vi "Assign DRT values from string.vi"(1 "Syntax":enum16{"GCS 1.0", "GCS 2.0"}(ring), 2 "Queried axes":string[](array[string]), 3 "Parameter no.":i32[](array[numeric]), 4 "Input string":string, 5 "error in":errorcluster, 6 "Parameter no. (hex)":u32[](array[numeric]) format="%.0x", 7 "Parameter no. format \n(Decimal: FALSE)":bool) -> (11 "Parameter no. out":i32[](array[numeric]), 12 "Queried axes out":string[](array[string]), 13 "Parameter no. (hex) out":u32[](array[numeric]) format="%.0x", 14 "Parameter values":dbl[](array[numeric]) format="%.6f", 15 "Parameter strings":string[](array[string]), 19 "error out":errorcluster)   [LabVIEW 2020]
doc: "This VI assigns numerical values / strings from input string to queried axes and parameter numbers. Sub-VI for DRT?.vi."
panel:
  # "This vi assigns values/strings from input string to queried axes and parameter numbers."
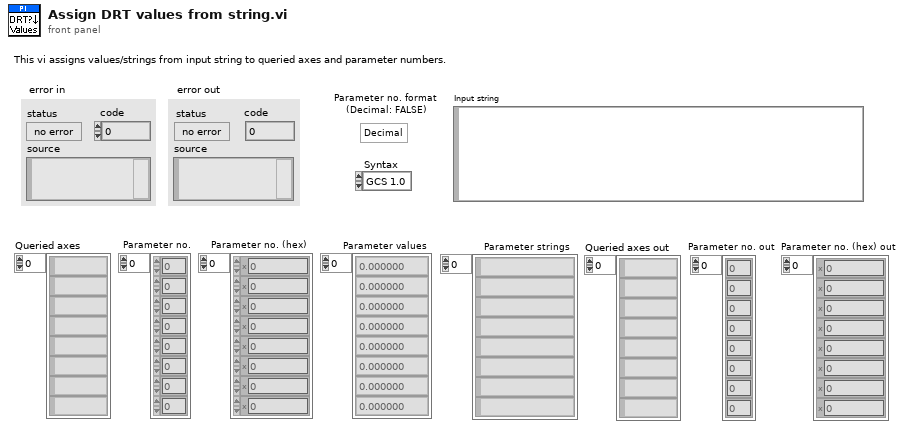
[diagram p1: front panel]
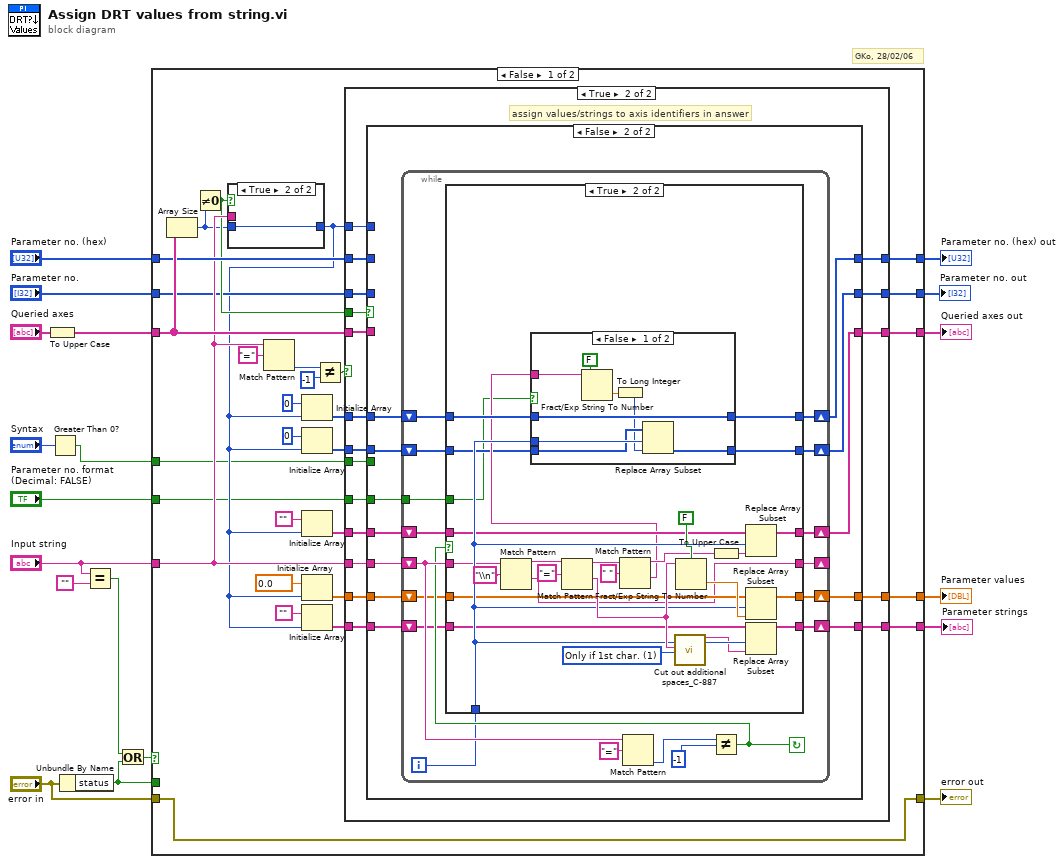
[diagram p0: block diagram]
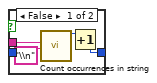
[diagram p2: hidden frame]
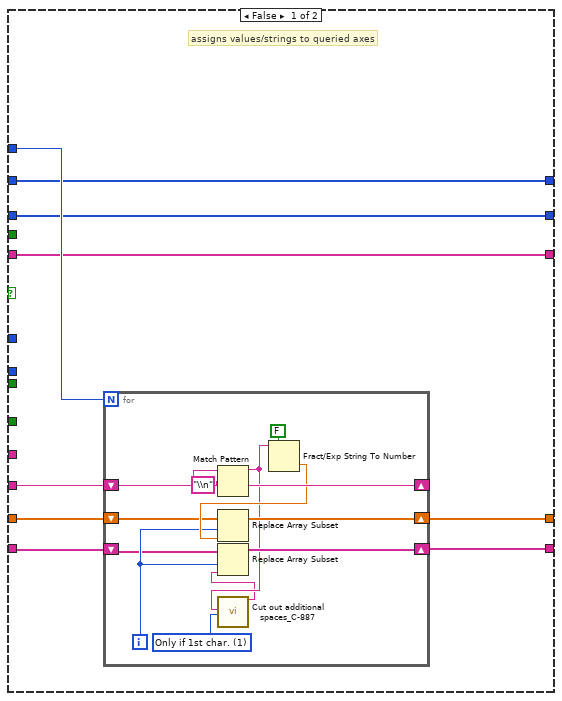
[diagram p3: hidden frame]
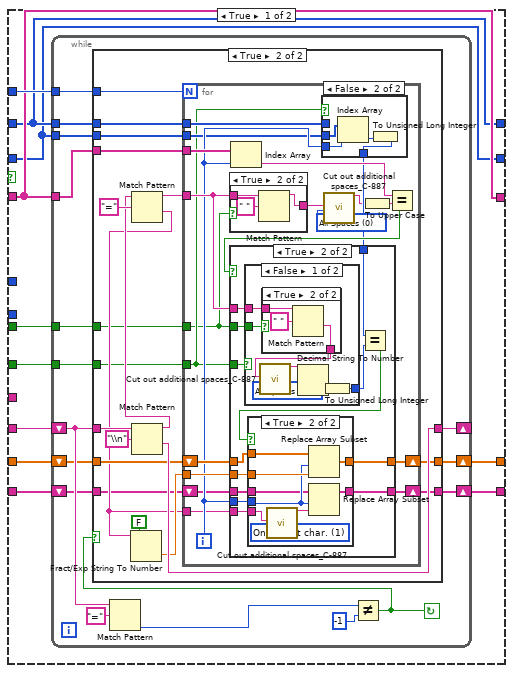
[diagram p4: hidden frame]
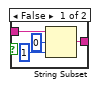
[diagram p6: hidden frame]
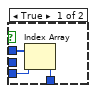
[diagram p7: hidden frame]
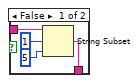
[diagram p9: hidden frame]
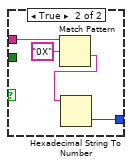
[diagram p10: hidden frame]
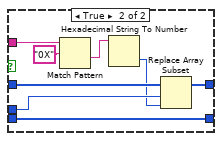
[diagram p13: hidden frame]
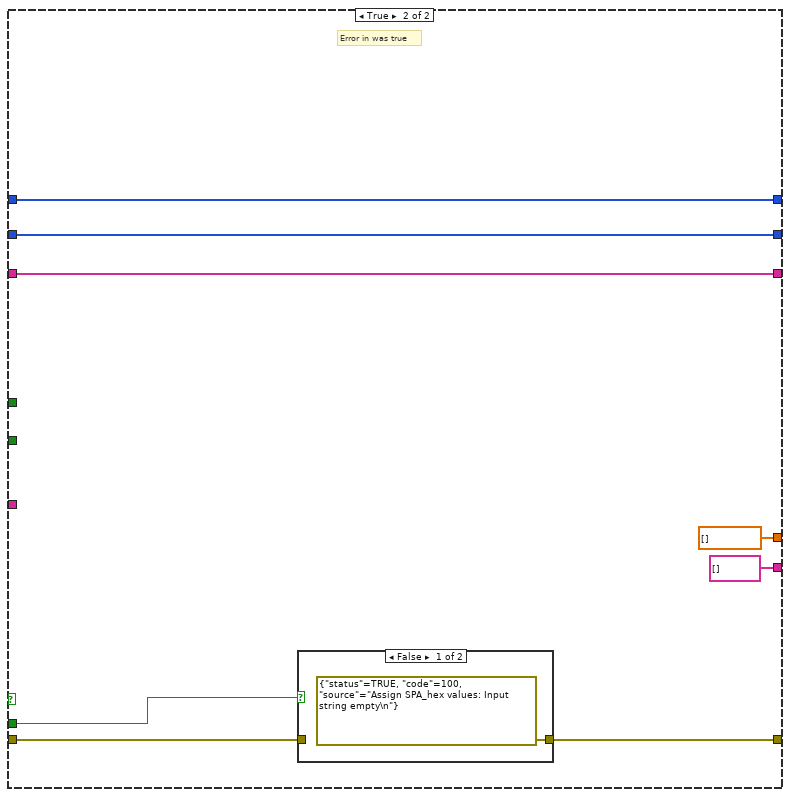
[diagram p14: hidden frame]
diagram:
  # "GKo, 28/02/06"
  n1 = To Upper Case(1:"Queried axes") -> (0:w12:string[])
  n2 = Greater Than 0?(x="Syntax") -> (x > 0?=w1:bool)
  n3 = Unbundle By Name("error in") -> ("status"=w9:bool)
  n4 = Equal?(x="Input string", y="") -> (x = y?=w10:bool)
  n5 = Or(x=w10, y=w9) -> (x .or. y?=w13:bool)
  n6 = case shown="False" w13 {
    tunnel: "Input string" -> [w34 _]
    tunnel: [w48 dbl[] [] ("Step Size")] -> w19
    tunnel: w12 -> [w47 w302]
    tunnel: [w20 w305] -> w16
    tunnel: "error in" -> [w20 w306]
    tunnel: "Parameter no. (hex)" -> [w40 w301]
    tunnel: w9 -> [_ w304]
    tunnel: [w37 string[] []] -> w8
    tunnel: [w29 w302] -> w7
    tunnel: [w28 w301] -> w6
    tunnel: "Parameter no." -> [w27 w300]
    tunnel: [w26 w300] -> w4
    tunnel: "Parameter no. format \n(Decimal: FALSE)" -> [w22 _]
    tunnel: w1 -> [w21 _]
    frame False {
      n7 = Array Size(array=w47) -> (size(s)=w30:i32)
      n8 = Not Equal To 0?(x=w30) -> (x != 0?=w33:bool)
      n9 = case shown="True" w33 {
        tunnel: [w49 w53] -> w24
        tunnel: w30 -> [_ w53]
        tunnel: w34 -> [w52 _]
        frame False {
          n10 = call "Count occurrences in string.vi"("Input string"=w52, "Expression"="\\n") -> ("Occurrences"=w50:i32)  [unwired: 17 out]
          n11 = Increment(x=w50) -> (x+1=w49:i32)
        }
        frame True {
        }
      }
      n12 = Match Pattern(string=w34, regular expression="=") -> (offset past match=w44:i32)  [unwired: 4 out]
      n13 = Initialize Array(u32 0 ("Element Data"), w24) -> (w31:u32[])
      n14 = Initialize Array(0 ("Element Data"), w24) -> (w23:i32[])
      n15 = Initialize Array("" ("Element Data"), w24) -> (w32:string[])
      n16 = Initialize Array(0.0 ("Element Data"), w24) -> (w41:dbl[])
      n17 = Initialize Array("" ("Element Data"), w24) -> (w38:string[])
      n18 = Not Equal?(x=w44, y=-1) -> (x != y?=w43:bool)
      n19 = case shown="True" w43 {
        tunnel: [w62 w92] -> w48
        tunnel: w34 -> [w61 w93]
        tunnel: w47 -> [w56 w91]
        tunnel: w41 -> [w60 w89]
        tunnel: w24 -> [w59 w90]
        tunnel: w40 -> [w55 w88]
        tunnel: w38 -> [w57 w87]
        tunnel: [w58 w86] -> w37
        tunnel: w33 -> [_ w85]
        tunnel: w32 -> [_ w84]
        tunnel: w31 -> [_ w83]
        tunnel: [w56 w82] -> w29
        tunnel: [w55 w81] -> w28
        tunnel: w27 -> [w54 w80]
        tunnel: [w54 w79] -> w26
        tunnel: w23 -> [_ w78]
        tunnel: w22 -> [_ w77]
        tunnel: w21 -> [_ w76]
        frame False {
          # "assigns values/strings to queried axes"
          n20 = for {
            N: w59 -> [_]
            shift-right: [w69] -> w62
            shift-left: w60 -> [w70]
            shift-right: [w74] -> _
            shift-left: w61 -> [w75]
            shift-right: [w68] -> w58
            shift-left: w57 -> [w66]
            i -> [w67]
            w63 = u16 1 items=["All Spaces", "Only if 1st char.", "Only if last char.", "Only if near \"=\""] ("Mode")
            n21 = Match Pattern(string=w75, regular expression="\\n") -> (before substring=w65:string, after substring=w74:string)  [unwired: 3 out]
            n22 = call "Cut out additional spaces_C-887.vi"("String"=w65, "Mode"=w63) -> ("String out"=w64:string)  [unwired: 17 out]
            n23 = Replace Array Subset(array=w66, new element=w64, index=w67) -> (w68:string[])
            n24 = Fract/Exp String To Number(use system decimal point (T)=FALSE, string=w65) -> (number=w71:dbl)  [unwired: 3 out]
            n25 = Replace Array Subset(array=w70, new element=w71, index=w67) -> (w69:dbl[])
          }
        }
        frame True {
          # "assign values/strings to axis identifiers in answer"
          n26 = case shown="False" w85 {
            tunnel: w93 -> [w104 w232]
            tunnel: [w103 w231] -> w92
            tunnel: w91 -> [w98 _]
            tunnel: w90 -> [w102 _]
            tunnel: w89 -> [w101 w230]
            tunnel: w88 -> [w97 _]
            tunnel: w87 -> [w100 w229]
            tunnel: [w99 w228] -> w86
            tunnel: w84 -> [_ w227]
            tunnel: w83 -> [_ w224]
            tunnel: [w98 w226] -> w82
            tunnel: [w97 w225] -> w81
            tunnel: w80 -> [w96 _]
            tunnel: [w96 w223] -> w79
            tunnel: w78 -> [_ w222]
            tunnel: w77 -> [w95 w221]
            tunnel: w76 -> [w94 _]
            frame True {
              n27 = while {
                shift-left: w100 -> [w108]
                shift-right: [w109] -> w99
                tunnel: w97 -> [w110]
                tunnel: w102 -> [w111]
                tunnel: w98 -> [w112]
                shift-left: w101 -> [w114]
                shift-right: [w113] -> w103
                shift-left: w104 -> [w117]
                shift-right: [w116] -> _
                tunnel: w96 -> [w107]
                tunnel: w95 -> [w106]
                tunnel: w94 -> [w105]
                stop <- w115 continue-if-true
                n28 = Match Pattern(string=w117, regular expression="=") -> (offset past match=w118:i32)  [unwired: 4 out]
                n29 = Not Equal?(x=w118, y=-1) -> (x != y?=w115:bool)
                n30 = case shown="True" w115 {
                  tunnel: w117 -> [w123 w141]
                  tunnel: [w123 w140] -> w116
                  tunnel: [w122 w138] -> w113
                  tunnel: w114 -> [w122 w139]
                  tunnel: w112 -> [_ w133]
                  tunnel: w111 -> [_ w130]
                  tunnel: w110 -> [_ w131]
                  tunnel: [w121 w128] -> w109
                  tunnel: w108 -> [w121 w127]
                  tunnel: w107 -> [_ w126]
                  tunnel: w106 -> [_ w125]
                  tunnel: w105 -> [_ w124]
                  frame False {
                  }
                  frame True {
                    n31 = Match Pattern(string=w141, regular expression="\\n") -> (before substring=w135:string, after substring=w140:string)  [unwired: 3 out]
                    n32 = Match Pattern(string=w135, regular expression="=") -> (before substring=w132:string, after substring=w129:string)  [unwired: 3 out]
                    n33 = Fract/Exp String To Number(use system decimal point (T)=FALSE, string=w129) -> (number=w134:dbl)  [unwired: 3 out]
                    n34 = for {
                      N: w130 -> [_]
                      tunnel: w134 -> [w162]
                      shift-right: [w160] -> w138
                      shift-left: w139 -> [w161]
                      tunnel: w133 -> [w159]
                      tunnel: w132 -> [w156]
                      tunnel: w131 -> [w155]
                      tunnel: w129 -> [w152]
                      shift-right: [w150] -> w128
                      shift-left: w127 -> [w151]
                      tunnel: w126 -> [w149]
                      tunnel: w125 -> [w148]
                      tunnel: w124 -> [w147]
                      i -> [w154]
                      w145 = u16 0 items=["All Spaces", "Only if 1st char.", "Only if last char.", "Only if near \"=\""] ("Mode")
                      n35 = case shown="True" w147 {
                        tunnel: [w164 w169] -> w146
                        tunnel: w156 -> [w163 w167]
                        frame False {
                          n36 = String Subset(string=w163, offset (0)=0, length (rest)=1 ("length")) -> (substring=w164:string)
                        }
                        frame True {
                          n37 = Match Pattern(string=w167, regular expression=" ") -> (before substring=w169:string)  [unwired: 4 out]
                        }
                      }
                      n38 = Index Array(array=w159, index=w154) -> (element=w158:string)
                      n39 = case shown="False" w148 {
                        tunnel: w155 -> [w172 _]
                        tunnel: w154 -> [w171 w176]
                        tunnel: [w170 w173] -> w153
                        tunnel: w149 -> [_ w174]
                        frame True {
                          n40 = Index Array(array=w172, index=w171) -> (element=w170:u32)
                        }
                        frame False {
                          n41 = Index Array(array=w174, index=w176) -> (element=w175:i32)
                          n42 = To Unsigned Long Integer(number=w175) -> (unsigned 32bit integer=w173:u32)
                        }
                      }
                      n43 = call "Cut out additional spaces_C-887.vi"("String"=w146, "Mode"=w145) -> ("String out"=w144:string)  [unwired: 17 out]
                      n44 = To Upper Case(1:w144) -> (0:w143:string)
                      n45 = Equal?(x=w158, y=w143) -> (x = y?=w157:bool)
                      n46 = case shown="True" w157 {
                        tunnel: w162 -> [_ w191]
                        tunnel: w154 -> [_ w188]
                        tunnel: w161 -> [w178 w190]
                        tunnel: [w178 w189] -> w160
                        tunnel: w156 -> [_ w187]
                        tunnel: w153 -> [_ w186]
                        tunnel: w152 -> [_ w183]
                        tunnel: w151 -> [w177 w182]
                        tunnel: [w177 w181] -> w150
                        tunnel: w148 -> [_ w180]
                        tunnel: w147 -> [_ w179]
                        frame False {
                        }
                        frame True {
                          n47 = case shown="False" w180 {
                            tunnel: w187 -> [w197 w209]
                            tunnel: [w192 w208] -> w185
                            tunnel: w179 -> [w196 _]
                            frame False {
                              w193 = u16 0 items=["All Spaces", "Only if 1st char.", "Only if last char.", "Only if near \"=\""] ("Mode")
                              n48 = case shown="True" w196 {
                                tunnel: [w200 w203] -> w195
                                tunnel: w197 -> [w199 w205]
                                frame False {
                                n49 = String Subset(string=w199, offset (0)=1, length (rest)=5 ("length")) -> (substring=w200:string)
                                }
                                frame True {
                                n50 = Match Pattern(string=w205, regular expression=" ") -> (after substring=w203:string)  [unwired: 4 out]
                                }
                              }
                              n51 = call "Cut out additional spaces_C-887.vi"("String"=w195, "Mode"=w193) -> ("String out"=w194:string)  [unwired: 17 out]
                              n52 = Decimal String To Number(string=w194) -> (number=w198:i32)  [unwired: 3 out]
                              n53 = To Unsigned Long Integer(number=w198) -> (unsigned 32bit integer=w192:u32)
                            }
                            frame True {
                              n54 = Match Pattern(string=w209, regular expression="0X") -> (after substring=w206:string)  [unwired: 4 out]
                              n55 = Hexadecimal String To Number(string=w206) -> (number=w208:u32)  [unwired: 3 out]
                            }
                          }
                          n56 = Equal?(x=w186, y=w185) -> (x = y?=w184:bool)
                          n57 = case shown="True" w184 {
                            tunnel: w191 -> [_ w220]
                            tunnel: w190 -> [w211 w219]
                            tunnel: [w211 w218] -> w189
                            tunnel: w188 -> [_ w217]
                            tunnel: w183 -> [_ w214]
                            tunnel: w182 -> [w210 w216]
                            tunnel: [w210 w215] -> w181
                            frame False {
                            }
                            frame True {
                              w212 = u16 1 items=["All Spaces", "Only if 1st char.", "Only if last char.", "Only if near \"=\""] ("Mode")
                              n58 = call "Cut out additional spaces_C-887.vi"("String"=w214, "Mode"=w212) -> ("String out"=w213:string)  [unwired: 17 out]
                              n59 = Replace Array Subset(array=w219, new element=w220, index=w217) -> (w218:dbl[])
                              n60 = Replace Array Subset(array=w216, new element=w213, index=w217) -> (w215:string[])
                            }
                          }
                        }
                      }
                    }
                  }
                }
              }
            }
            frame False {
              n61 = while {
                shift-left: w227 -> [w239]
                shift-right: [w236] -> w226
                shift-left: w224 -> [w238]
                shift-right: [w237] -> w225
                shift-left: w229 -> [w241]
                shift-right: [w242] -> w228
                shift-left: w230 -> [w244]
                shift-right: [w243] -> w231
                shift-left: w232 -> [w247]
                shift-right: [w246] -> _
                shift-right: [w234] -> w223
                shift-left: w222 -> [w235]
                tunnel: w221 -> [w233]
                i -> [w240]
                stop <- w245 continue-if-true
                n62 = Match Pattern(string=w247, regular expression="=") -> (offset past match=w248:i32)  [unwired: 4 out]
                n63 = Not Equal?(x=w248, y=-1) -> (x != y?=w245:bool)
                n64 = case shown="True" w245 {
                  tunnel: w247 -> [w256 w267]
                  tunnel: [w256 w266] -> w246
                  tunnel: [w255 w273] -> w243
                  tunnel: w244 -> [w255 w269]
                  tunnel: [w254 w274] -> w242
                  tunnel: w241 -> [w254 w268]
                  tunnel: w240 -> [_ w272]
                  tunnel: w239 -> [w252 w271]
                  tunnel: w238 -> [w253 w270]
                  tunnel: [w253 w265] -> w237
                  tunnel: [w252 w263] -> w236
                  tunnel: w235 -> [w251 w262]
                  tunnel: [w251 w261] -> w234
                  tunnel: w233 -> [_ w260]
                  frame False {
                  }
                  frame True {
                    w258 = u16 1 items=["All Spaces", "Only if 1st char.", "Only if last char.", "Only if near \"=\""] ("Mode")
                    n65 = Match Pattern(string=w267, regular expression="\\n") -> (before substring=w280:string, after substring=w266:string)  [unwired: 3 out]
                    n66 = Match Pattern(string=w280, regular expression="=") -> (before substring=w277:string, after substring=w278:string)  [unwired: 3 out]
                    n67 = Match Pattern(string=w277, regular expression=" ") -> (before substring=w275:string, after substring=w264:string)  [unwired: 3 out]
                    n68 = case shown="False" w260 {
                      tunnel: w272 -> [w288 w299]
                      tunnel: w270 -> [w291 w298]
                      tunnel: [w291 w297] -> w265
                      tunnel: w264 -> [w285 w295]
                      tunnel: w262 -> [w287 w292]
                      tunnel: [w286 w292] -> w261
                      frame False {
                        n69 = Fract/Exp String To Number(use system decimal point (T)=FALSE, string=w285) -> (number=w289:dbl)  [unwired: 3 out]
                        n70 = To Long Integer(number=w289) -> (32bit integer=w284:i32)
                        n71 = Replace Array Subset(array=w287, new element=w284, index=w288) -> (w286:i32[])
                      }
                      frame True {
                        n72 = Match Pattern(string=w295, regular expression="0X") -> (after substring=w294:string)  [unwired: 4 out]
                        n73 = Hexadecimal String To Number(string=w294) -> (number=w293:u32)  [unwired: 3 out]
                        n74 = Replace Array Subset(array=w298, new element=w293, index=w299) -> (w297:u32[])
                      }
                    }
                    n75 = call "Cut out additional spaces_C-887.vi"("String"=w278, "Mode"=w258) -> ("String out"=w259:string)  [unwired: 17 out]
                    n76 = Fract/Exp String To Number(use system decimal point (T)=FALSE, string=w278) -> (number=w279:dbl)  [unwired: 3 out]
                    n77 = To Upper Case(1:w275) -> (0:w257:string)
                    n78 = Replace Array Subset(array=w271, new element=w257, index=w272) -> (w263:string[])
                    n79 = Replace Array Subset(array=w269, new element=w279, index=w272) -> (w273:dbl[])
                    n80 = Replace Array Subset(array=w268, new element=w259, index=w272) -> (w274:string[])
                  }
                }
              }
            }
          }
        }
      }
    }
    frame True {
      # "Error in was true"
      n81 = case shown="False" w304 {
        tunnel: w306 -> [_ w309]
        tunnel: [errorcluster {"status"=TRUE, "code"=100, "source"="Assign SPA_hex values: Input string empty\n"} ("error out") w309] -> w305
        frame False {
        }
        frame True {
        }
      }
    }
  }
  "Parameter values" <- w19
  "error out" <- w16
  "Parameter strings" <- w8
  "Parameter no. (hex) out" <- w6
  "Queried axes out" <- w7
  "Parameter no. out" <- w4
